vi "AdvBGSub_Bella.vi"(8 "error in":errorcluster, 11 "Refnum in":T2) -> (0 "error out":errorcluster, 2 "-x":sgl, 3 "Refnum out":T2, 4 "empty image":bool)   [LabVIEW 2020]
uses:
  IMAQ Image.ctl
  NI_Vision_Development_Module.lvlib
panel:
  out "Histogram Report":T1 {"Standard  Variation" format="%.2f"; "Mean Value" format="%.2f"; "Interval Width" format="%.2f"; "Starting Value" format="%.2f"; "Maximal Value" format="%.2f"; "Minimal Value" format="%.2f"}
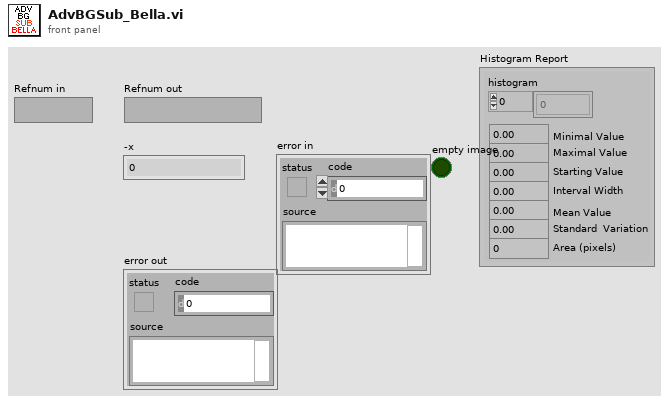
[diagram p1: front panel]
types:
  T1 = cluster{"histogram":u32[], "Minimal Value":sgl, "Maximal Value":sgl, "Starting Value":sgl, "Interval Width":sgl, "Mean Value":sgl, "Standard  Variation":sgl, "Area (pixels)":i32}
  T2 = typedef "IMAQ Image.ctl" = refnum<image>
  T3 = typedef "Image Type" = u32
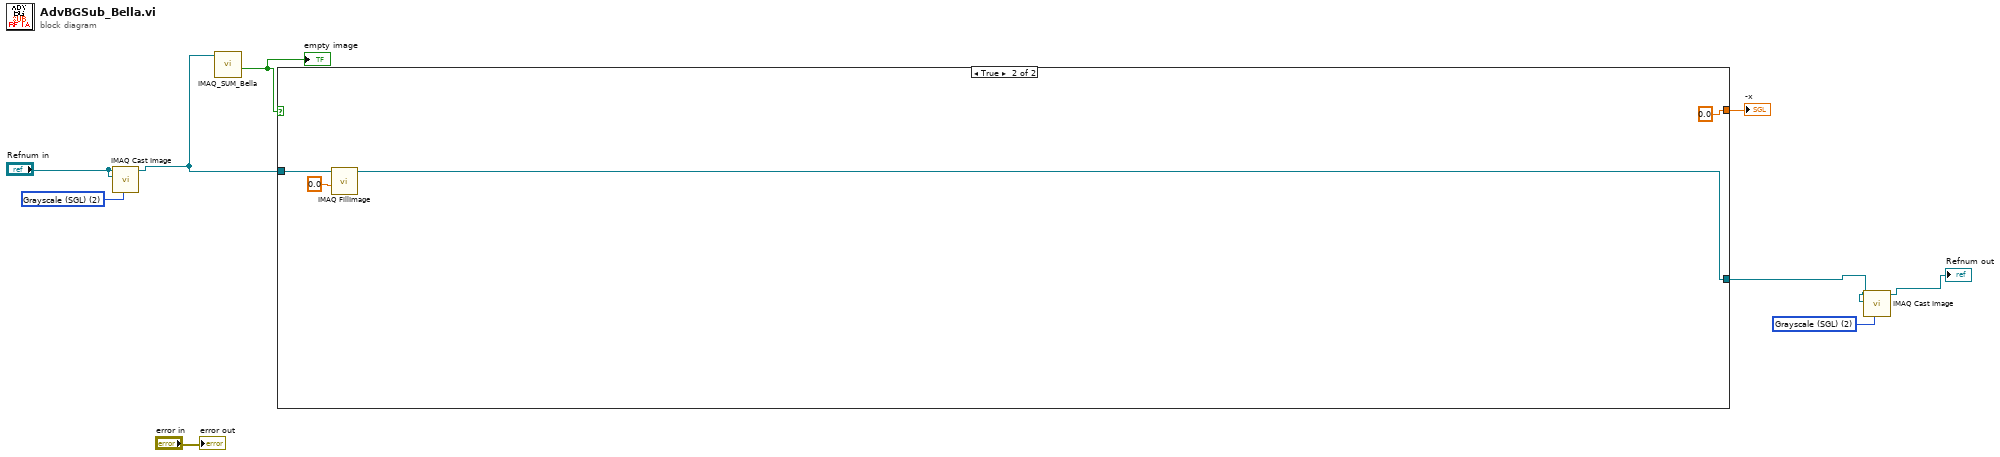
[diagram p0: block diagram]
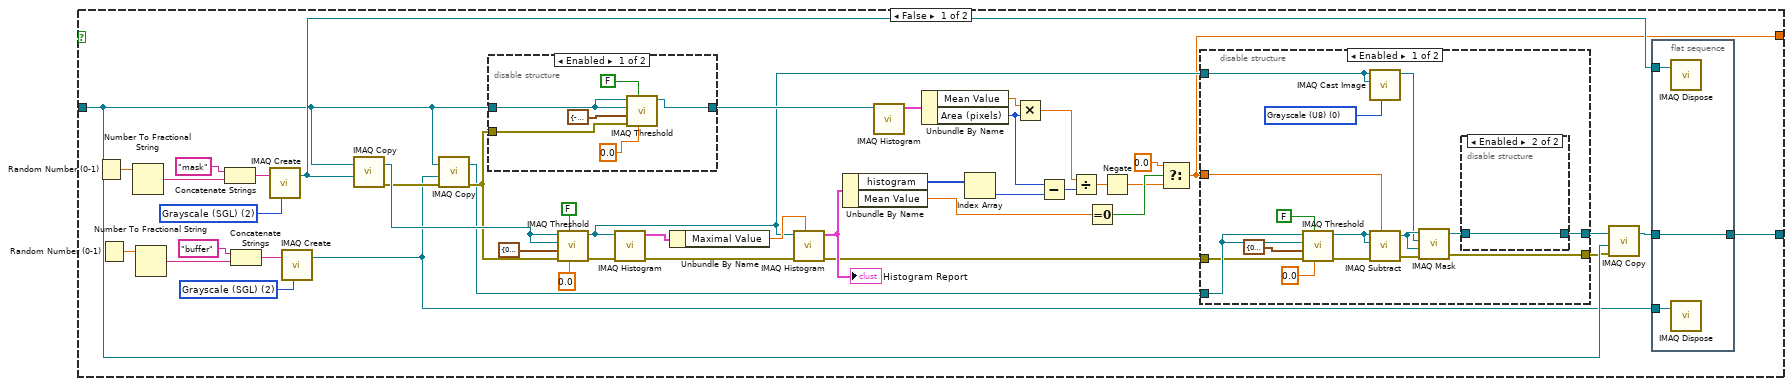
[diagram p2: hidden frame]
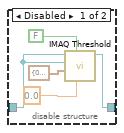
[diagram p4: hidden frame]
diagram:
  w5 = T3 2 items=["Grayscale (U8)", "Grayscale (I16)", "Grayscale (SGL)", "Complex (CSG)", "RGB (U32)", "HSL (U32)", "RGB (U64)", "Grayscale (U16)"] ("Image Type")
  w6 = T3 2 items=["Grayscale (U8)", "Grayscale (I16)", "Grayscale (SGL)", "Complex (CSG)", "RGB (U32)", "HSL (U32)", "RGB (U64)", "Grayscale (U16)"] ("Image Type")
  n1 = call "IMAQ Cast Image"("Image Type"=w6, "Image Dst"="Refnum in", "Image Src"="Refnum in") -> ("Image Dst Out"=w2:T2)  [unwired: 7 in, 1 out]
  n2 = call "IMAQ_SUM_Bella.vi"("Image"=w2) -> ("empty Image"=w1:bool)  [unwired: 8 in, 2 out]
  "empty image" <- w1
  n3 = case shown="True" w1 {
    tunnel: w2 -> [w22 w89]
    tunnel: [w21 w88] -> w4
    tunnel: [w19 sgl 0.0] -> w8
    frame False {
      w29 = T3 2 items=["Grayscale (U8)", "Grayscale (I16)", "Grayscale (SGL)", "Complex (CSG)", "RGB (U32)", "HSL (U32)", "RGB (U64)", "Grayscale (U16)"] ("Image Type")
      w34 = T3 2 items=["Grayscale (U8)", "Grayscale (I16)", "Grayscale (SGL)", "Complex (CSG)", "RGB (U32)", "HSL (U32)", "RGB (U64)", "Grayscale (U16)"] ("Image Type")
      n4 = Random Number (0-1)() -> (number: 0 to 1=w36:dbl)
      n5 = Random Number (0-1)() -> (number: 0 to 1=w32:dbl)
      n6 = Number To Fractional String(number=w36) -> (F-format string=w38:string)  [unwired: 3 in]
      n7 = Number To Fractional String(number=w32) -> (F-format string=w30:string)  [unwired: 3 in]
      n8 = Concatenate Strings("mask" ("Image Name"), w38) -> (w35:string)
      n9 = Concatenate Strings("buffer" ("Image Name"), w30) -> (w33:string)
      n10 = call "IMAQ Create"("Image Name"=w35, "Image Type"=w34) -> ("New Image"=w28:T2)  [unwired: 3 in, 1 out]
      n11 = call "IMAQ Create"("Image Name"=w33, "Image Type"=w29) -> ("New Image"=w12:T2)  [unwired: 3 in, 1 out]
      n12 = call "IMAQ Copy"("Image Dst"=w28, "Image Src"=w22) -> ("error out"=w15:errorcluster, "Image Dst Out"=w50:T2)  [unwired: 4 in]
      n13 = call "IMAQ Copy"("error in (no error)"=w15, "Image Dst"=w12, "Image Src"=w22) -> ("error out"=w14:errorcluster, "Image Dst Out"=w11:T2)  [unwired: 3 in]
      n14 = disable-structure shown="Enabled" {
        disable-tunnel: [w60 w64] -> w41
        disable-tunnel: w22 -> [w59 w64]
        disable-tunnel: w14 -> [w58 _]
        frame Enabled {
          n15 = call "IMAQ Threshold"("Replace Value"=sgl 0.0, "Keep/Replace Value (Replace)"=FALSE, "error in (no error)"=w58, "Range"=cluster{"Lower value":sgl, "Upper value":sgl} {"Lower value"=-99999.0, "Upper value"=0.0}, "Image Dst"=w59, "Image Src"=w59) -> ("Image Dst Out"=w60:T2)  [unwired: 4 in, 1 out]
        }
        frame Disabled {
        }
      }
      n16 = call "IMAQ Threshold"("Replace Value"=sgl 0.0, "Keep/Replace Value (Replace)"=FALSE, "error in (no error)"=w14, "Range"=cluster{"Lower value":sgl, "Upper value":sgl} {"Lower value"=0.0, "Upper value"=99999.0}, "Image Dst"=w50, "Image Src"=w50) -> ("error out"=w16:errorcluster, "Image Dst Out"=w25:T2)  [unwired: 4 in]
      n17 = call "IMAQ Histogram"("error in (no error)"=w16, "Image"=w25) -> ("error out"=w13:errorcluster, "Histogram Report"=w49:T1)  [unwired: 8 in]
      n18 = Unbundle By Name(w49) -> ("Maximal Value"=w43:sgl)
      n19 = call "IMAQ Histogram"("Number of Classes"=w43, "error in (no error)"=w13, "Image"=w25) -> ("error out"=w17:errorcluster, "Histogram Report"=w47:T1)  [unwired: 7 in]
      "Histogram Report" <- w47
      n20 = Unbundle By Name(w47) -> ("histogram"=w46:u32[], "Mean Value"=w10:sgl)
      n21 = call "IMAQ Histogram"("Image"=w41) -> ("Histogram Report"=w48:T1)  [unwired: 9 in, 1 out]
      n22 = Unbundle By Name(w48) -> ("Mean Value"=w42:sgl, "Area (pixels)"=w39:i32)
      n23 = Index Array(array=w46) -> (element=w45:u32)  [unwired: 1 in]
      n24 = Multiply(x=w42, y=w39) -> (x*y=w40:sgl)
      n25 = Subtract(x=w39, y=w45) -> (x-y=w44:u32)
      n26 = Divide(x=w40, y=w44) -> (x/y=w54:sgl)
      n27 = Equal To 0?(x=w10) -> (x = 0?=w24:bool)
      n28 = Negate(x=w54) -> (-x=w20:sgl)
      n29 = Select(t=0.0, s=w24, f=w20) -> (s? t:f=w19:dbl)
      n30 = disable-structure shown="Enabled" {
        disable-tunnel: w19 -> [w80 _]
        disable-tunnel: [w79 w87] -> w27
        disable-tunnel: w11 -> [w76 w87]
        disable-tunnel: w25 -> [w70 _]
        disable-tunnel: [w67 _] -> w18
        disable-tunnel: w17 -> [w65 _]
        frame Enabled {
          w69 = T3 0 items=["Grayscale (U8)", "Grayscale (I16)", "Grayscale (SGL)", "Complex (CSG)", "RGB (U32)", "HSL (U32)", "RGB (U64)", "Grayscale (U16)"] ("Image Type")
          n31 = call "IMAQ Threshold"("Replace Value"=sgl 0.0, "Keep/Replace Value (Replace)"=FALSE, "error in (no error)"=w65, "Range"=cluster{"Lower value":sgl, "Upper value":sgl} {"Lower value"=0.0, "Upper value"=9999999.0}, "Image Dst"=w76, "Image Src"=w76) -> ("error out"=w66:errorcluster, "Image Dst Out"=w74:T2)  [unwired: 4 in]
          n32 = call "IMAQ Cast Image"("Image Type"=w69, "Image Dst"=w70, "Image Src"=w70) -> ("Image Dst Out"=w68:T2)  [unwired: 7 in, 1 out]
          n33 = call "IMAQ Subtract"("Image Src A"=w74, "Constant"=w80, "Image Dst"=w74, "error in (no error)"=w66) -> ("Image Dst Out"=w72:T2, "error out"=w73:errorcluster)  [unwired: 3 in]
          n34 = call "IMAQ Mask"("error in (no error)"=w73, "Image Dst"=w72, "Image Mask"=w68, "Image Src"=w72) -> ("error out"=w67:errorcluster, "Image Dst Out"=w71:T2)  [unwired: 1 in]
          n35 = disable-structure shown="Enabled" {
            disable-tunnel: [w82 w86] -> w79
            disable-tunnel: w71 -> [w81 w86]
            frame Disabled {
              n36 = call "IMAQ Threshold"("Replace Value"=sgl 0.0, "Keep/Replace Value (Replace)"=FALSE, "Range"=cluster{"Lower value":sgl, "Upper value":sgl} {"Lower value"=0.0, "Upper value"=9999999.0}, "Image Dst"=w81, "Image Src"=w81) -> ("Image Dst Out"=w82:T2)  [unwired: 5 in, 1 out]
            }
            frame Enabled {
            }
          }
        }
        frame Disabled {
        }
      }
      n37 = call "IMAQ Copy"("error in (no error)"=w18, "Image Dst"=w22, "Image Src"=w27) -> ("Image Dst Out"=w26:T2)  [unwired: 3 in, 1 out]
      n38 = flat-sequence {
        tunnel: w26 -> [w56]
        tunnel: w28 -> [w57]
        tunnel: [w56] -> w21
        tunnel: w12 -> [w55]
        frame #0 {
          n39 = call "IMAQ Dispose"("Image"=w57) -> ()  [unwired: 5 in, 1 out]
          n40 = call "IMAQ Dispose"("Image"=w55) -> ()  [unwired: 5 in, 1 out]
        }
      }
    }
    frame True {
      n41 = call "IMAQ FillImage"("Pixel Value (U8, U16, I16, Float)"=sgl 0.0, "Image"=w89) -> ("Image Out"=w88:T2)  [unwired: 8 in, 1 out]
    }
  }
  "-x" <- w8
  n42 = call "IMAQ Cast Image"("Image Type"=w5, "Image Dst"=w4, "Image Src"=w4) -> ("Image Dst Out"=→"Refnum out":T2)  [unwired: 7 in, 1 out]
  "error out" <- "error in"
